vi "Block-Down-Upload.vi"() -> ()   [LabVIEW 2020]
uses:
  lib/Snap7.lvlib
panel:
  out "Download Status":string="No Error"
  in  "New Block Number":i32=1
  out "?":string
  in  "BlockType":i32(ring)=66 items=["OB"=56, "DB"=65, "SDB"=66, "FC"=67, "SFC"=68, "FB"=69, "SFB"=70]
  out "Size Get":i32
  out "Upload Status":string="No Error"
  in  "Number":i32=1
  in  "Slot":i32=2
  in  "Rack":i32
  in  "Address IP":string="192.168.1.12"
  # "Upload Block"
  # "Download Block"
  # "WARNING !!!\nThis program will overwrite\nthe New Block"
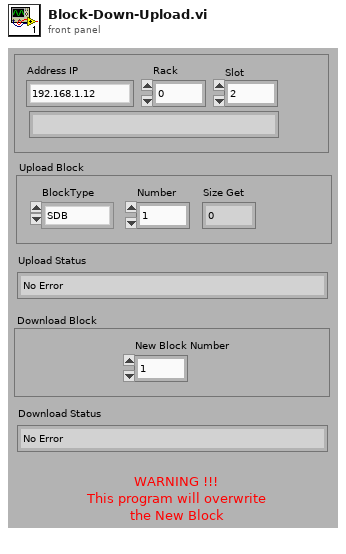
[diagram p1: front panel]
types:
  T1 = enum16{"big-endian, network order", "native, host order", "little-endian"}
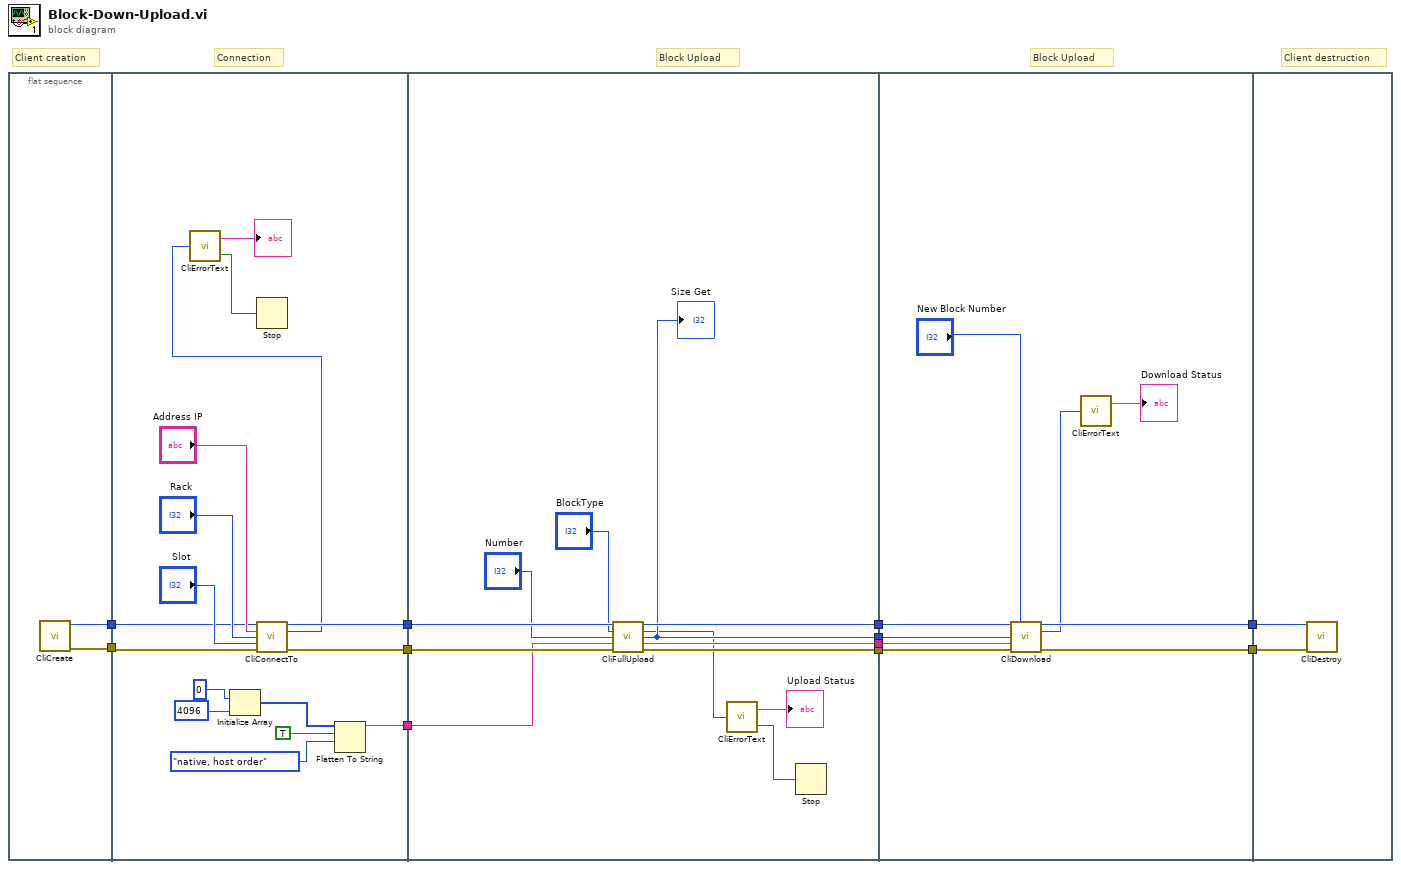
[diagram p0: block diagram]
diagram:
  # "Block Upload"
  # "Client destruction"
  # "Block Upload"
  # "Connection"
  # "Client creation"
  n1 = flat-sequence {
    tunnel: [w13] -> w8
    tunnel: [w12] -> w7
    tunnel: [w24] -> w11
    tunnel: [w17] -> w10
    tunnel: [w23] -> w9
    tunnel: w8 -> [w19]
    tunnel: w7 -> [w18]
    tunnel: w11 -> [w41]
    tunnel: w10 -> [w40]
    tunnel: w9 -> [w39]
    tunnel: [w38] -> w6
    tunnel: [w37] -> w4
    tunnel: [w36] -> w2
    tunnel: [w35] -> w1
    tunnel: w6 -> [w50]
    tunnel: [w48] -> w5
    tunnel: w4 -> [w49]
    tunnel: [w47] -> w3
    tunnel: w2 -> [w46]
    tunnel: w1 -> [w44]
    tunnel: w5 -> [w52]
    tunnel: w3 -> [w51]
    frame #0 {
      n2 = call "CliCreate.vi"() -> ("ref out"=w13:u64, "error out"=w12:errorcluster)  [unwired: 14 in]
    }
    frame #1 {
      n3 = Initialize Array(u8 0, 4096) -> (w27:u8[])
      n4 = call "CliConnectTo.vi"("ref in"=w19, "Address"="Address IP", "Rack"="Rack", "Slot"="Slot", "error in (no error)"=w18) -> ("ref out"=w17:u64, "Result"=w14:i32, "error out"=w24:errorcluster)  [unwired: 8 in]
      n5 = call "CliErrorText.vi"("ErrNo"=w14) -> ("Error"=w15:bool, "ErrMessage"=→"?":string)
      n6 = Stop(stop? (T)=w15) -> ()
      n7 = Flatten To String(anything=w27, prepend array or string size? (T)=TRUE, byte order (0:big-endian, network order)=T1."native, host order") -> (data string=w23:string)  [unwired: 1 in, 2 out]
    }
    frame #2 {
      n8 = call "CliFullUpload.vi"("ref in"=w40, "BlockType"="BlockType", "Block Number"="Number", "data in"=w39, "error in (no error)"=w41) -> ("ref out"=w38:u64, "Result"=w34:i32, "SizeGet"=w36:i32, "data out"=w35:string, "error out"=w37:errorcluster)  [unwired: 6 in]
      "Size Get" <- w36
      n9 = call "CliErrorText.vi"("ErrNo"=w34) -> ("Error"=w30:bool, "ErrMessage"=→"Upload Status":string)
      n10 = Stop(stop? (T)=w30) -> ()
    }
    frame #3 {
      n11 = call "CliDownload.vi"("ref in"=w50, "Block Number"="New Block Number", "Size"=w46, "data in"=w44, "error in (no error)"=w49) -> ("ref out"=w48:u64, "Result"=w42:i32, "error out"=w47:errorcluster)  [unwired: 8 in]
      n12 = call "CliErrorText.vi"("ErrNo"=w42) -> ("ErrMessage"=→"Download Status":string)  [unwired: 1 out]
    }
    frame #4 {
      n13 = call "CliDestroy.vi"("ref in"=w52, "error in (no error)"=w51) -> ()  [unwired: 13 in, 1 out]
    }
  }
